vi "ThresholdCore.vi"(6 "Threshold":u8, 7 "Max Value":u8, 8 "error in (no error)":errorcluster, 9 "Mode":T1[](array[typedef]), 10 "Threshold Result":refnum<data-value>, 11 "Greyscale Image-Source":refnum<data-value>) -> (0 "error out":errorcluster)   [LabVIEW 2020, in "g_ar_toolkit.image.lvlib"]
uses:
  g_ar_toolkit.image.lvlib
  Threshold Types.ctl
  g_ar_toolkit.common/g_ar_toolkit.common.lvlib
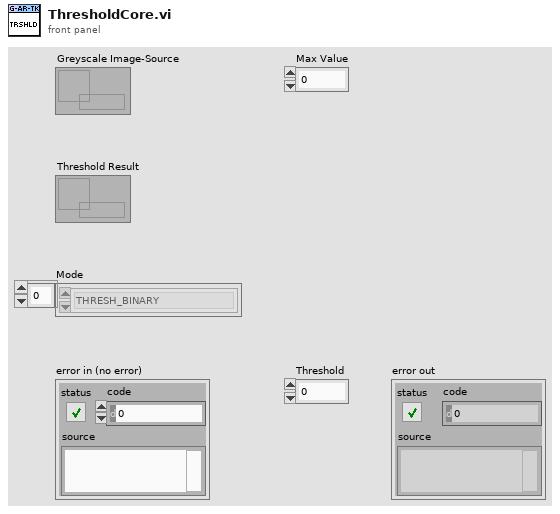
[diagram p1: front panel]
types:
  T1 = typedef "g_ar_toolkit.image.lvlib/Threshold Types.ctl" = enum8{"THRESH_BINARY", "THRESH_BINARY_INV", "THRESH_TRUNC", "THRESH_TOZERO", "THRESH_TOZERO_INV", "THRESH_MASK", "THRESH_OTSU", "THRESH_TRIANGLE"}
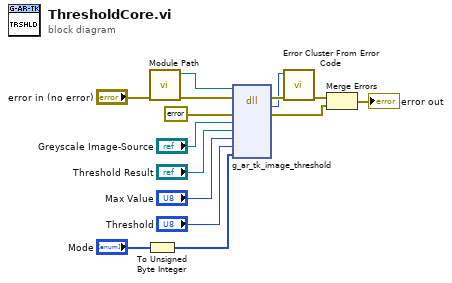
[diagram p0: block diagram]
diagram:
  n1 = To Unsigned Byte Integer(number="Mode") -> (unsigned 8bit integer=w3:u8[])
  n2 = call "Module Path.vi"("error in (no error)"="error in (no error)") -> ("error out"=w2:errorcluster, "Path"=w1:path)  [unwired: 9 in]
  n3 = dll-call lib="?" fn="g_ar_tk_image_threshold" ("g_ar_toolkit.*.*:g_ar_tk_image_in_range")(path in=w1, error in=w2, "error_cluster"=errorcluster {"status"=FALSE, "code"=0, "source"=""} ("error constant"), "EDVR src"="Greyscale Image-Source", "EDVR dst"="Threshold Result", "max_value"="Max Value", "threshold"="Threshold", "flags"=w3) -> (error out=w13:errorcluster, "MgErr"=w12:i32, "error_cluster"=w9:errorcluster)  [unwired: 6 in, 1 out]
  n4 = call <vilib>:"Error Cluster From Error Code.vi"("error in (no error)"=w13, "error code (0)"=w12) -> ("error out"=w11:errorcluster)  [unwired: 7 in]
  n5 = Merge Errors(w11, w9) -> (→"error out":errorcluster)
